vi "AMC Local Process 2.vi"() -> ()   [LabVIEW 2009]
uses:
  vi.lib/NI/AMC/AMC.lvlib
panel:
  in  "Process 1":bool
  out "Process":bool
  out "Status":string
  in  "Local Process":bool
  in  "Exit":bool
  in  "State Variables":cluster{"CurrentFile":path}
  # "Process 2"
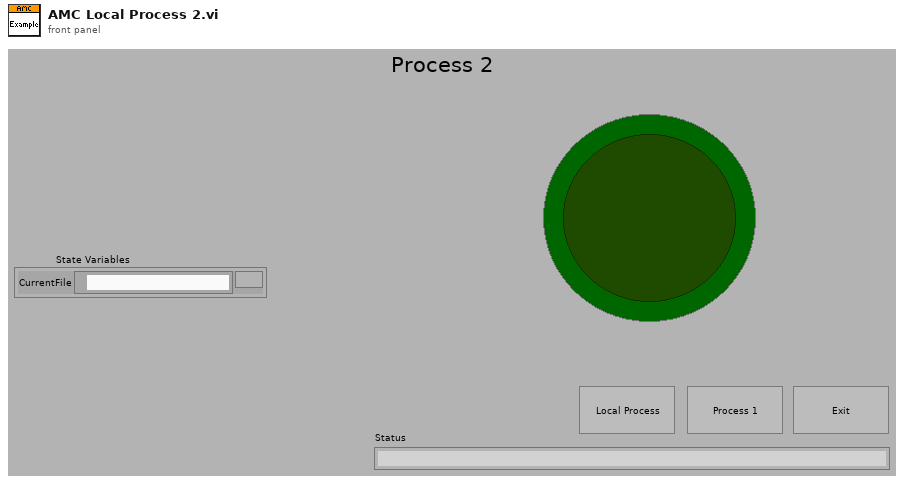
[diagram p1: front panel]
types:
  T1 = typedef "AMC.lvlib/Message Queue.ctl" = refnum<queue>
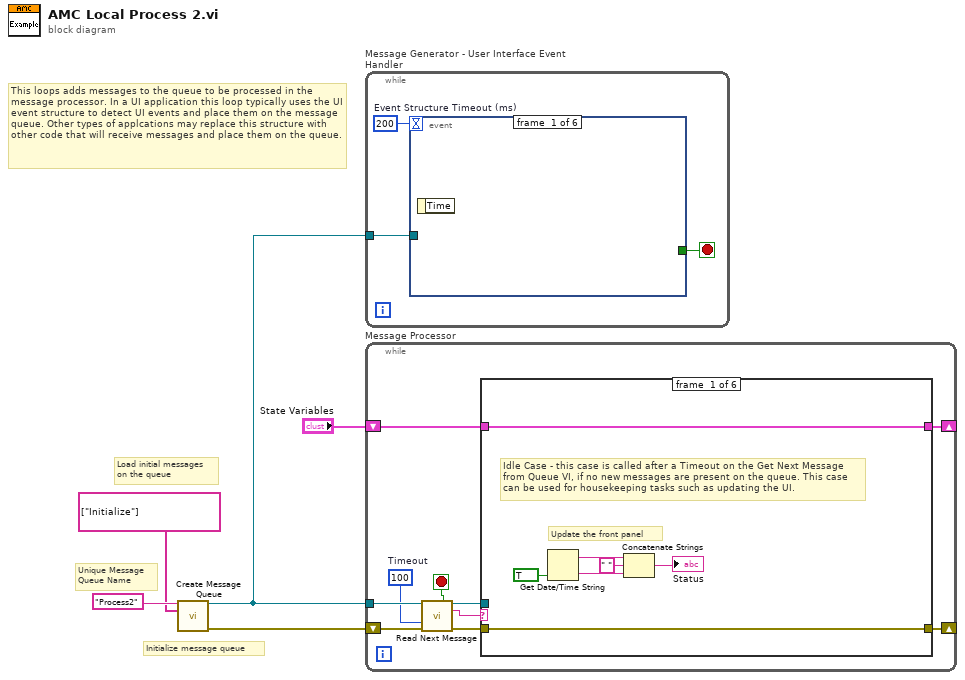
[diagram p0: block diagram]
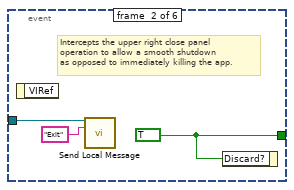
[diagram p2: hidden frame]
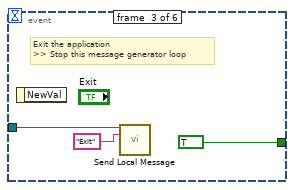
[diagram p3: hidden frame]
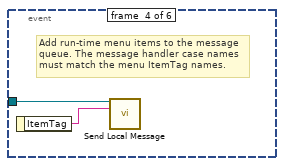
[diagram p4: hidden frame]
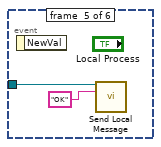
[diagram p5: hidden frame]
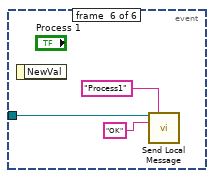
[diagram p6: hidden frame]
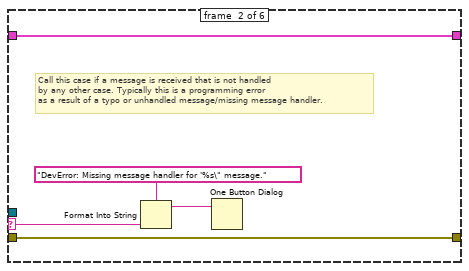
[diagram p7: hidden frame]
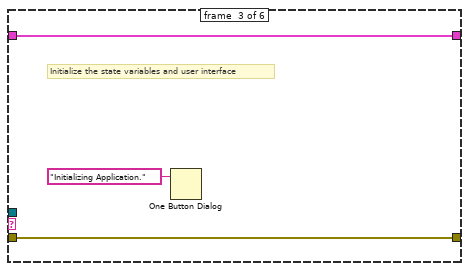
[diagram p8: hidden frame]
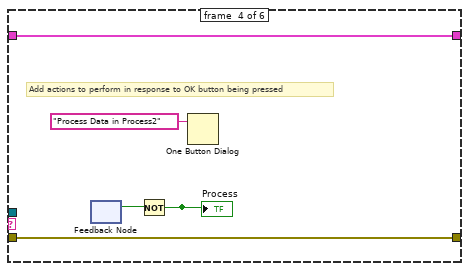
[diagram p9: hidden frame]
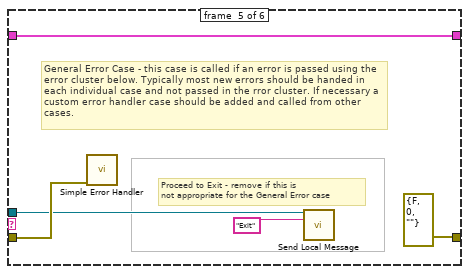
[diagram p10: hidden frame]
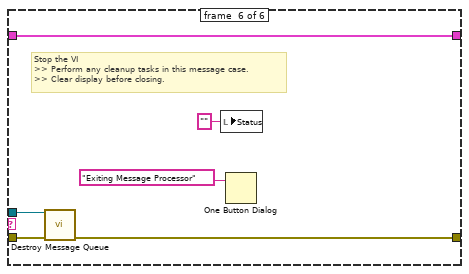
[diagram p11: hidden frame]
diagram:
  # "This loops adds messages to the queue to be processed in the message processor. In a UI application this loop typically uses the UI event structure to detect UI events and place them on the message queue. Other types of applcations may replace this structure with other code that will receive messages and place them on the queue."
  # "Initialize message queue"
  # "Unique Message\nQueue Name"
  # "Load initial messages\non the queue"
  n1 = call "Create Message Queue.vi"("message queue name"="Process2" ("Message queue name (unnamed)"), "initial message names"=string[] ["Initialize"]) -> ("message queue out"=w5:T1, "error out"=w3:errorcluster)  [unwired: 12 in]
  n2 = while "Message Generator - User Interface Event Handler" {
    tunnel: w5 -> [w6]
    stop <- w7 stop-if-true
    w8 = 200  # Event Structure Timeout (ms)
    n3 = event shown="[5] \"Process 1\": Value Change" {
      selector: _ -> [_ _ _ _ _ _]
      dyn-events: _ -> [_ _ _ _ _ _]
      timeout: w8 -> [_ _ _ _ _ _]
      tunnel: [_ w11 TRUE ("Discard?") _ _ _] -> w7
      tunnel: w6 -> [_ w10 w13 w16 w18 w21]
      event #0 {
        n4 = event-data() -> ()  [unwired: 2 out]
      }
      event #1 {
        w11 = TRUE ("Discard?")
        # "Intercepts the upper right close panel\noperation to allow a smooth shutdown\nas opposed to immediately killing the app."
        n5 = event-data() -> ()  [unwired: 2 out]
        n6 = call "Send Local Message.vi"("message queue in"=w10, "message name"="Exit") -> ()  [unwired: 11 in, 3 out]
        n7 = event-data("Discard?"=w11) -> ()  [unwired: 1 in, 1 out]
      }
      event #2 {
        # "Exit the application\n>> Stop this message generator loop"
        n8 = event-data() -> ()  [unwired: 2 out]
        n9 = call "Send Local Message.vi"("message queue in"=w13, "message name"="Exit") -> ()  [unwired: 11 in, 3 out]
      }
      event #3 {
        # "Add run-time menu items to the message\nqueue. The message handler case names must match the menu ItemTag names."
        n10 = event-data() -> ("ItemTag"=w15:string)  [unwired: 1 out]
        n11 = call "Send Local Message.vi"("message queue in"=w16, "message name"=w15) -> ()  [unwired: 11 in, 3 out]
      }
      event #4 {
        n12 = event-data() -> ()  [unwired: 2 out]
        n13 = call "Send Local Message.vi"("message queue in"=w18, "message name"="OK") -> ()  [unwired: 11 in, 3 out]
      }
      event #5 {
        n14 = event-data() -> ()  [unwired: 2 out]
        n15 = call "Send Local Message.vi"("message queue in"=w21, "receiver process (\"\" - local)"="Process1" ("process"), "message name"="OK") -> ()  [unwired: 10 in, 3 out]
      }
    }
  }
  n16 = while "Message Processor" {
    shift-left: w3 -> [w26]
    shift-right: [w27] -> _
    tunnel: w5 -> [w25]
    shift-left: "State Variables" -> [w31]
    shift-right: [w30] -> _
    stop <- w24 stop-if-true
    w22 = 100  # Timeout
    n17 = call "Read Next Message.vi"("message queue in"=w25, "timeout (1 ms)"=w22, "error in"=w26) -> ("exit process?"=w24:bool, "message queue out"=w29:T1, "message name"=w23:string, "error out"=w28:errorcluster)  [unwired: 5 in, 4 out]
    n18 = case shown="\"Initialize\"" w23 {
      selector: w23 -> [_ w41 _ _ _ _]
      tunnel: [w38 w43 w46 w50 w56 w61] -> w30
      tunnel: w31 -> [w38 w43 w46 w50 w56 w61]
      tunnel: w29 -> [_ _ _ _ w53 w58]
      tunnel: w28 -> [w37 w42 w45 w51 w54 w62]
      tunnel: [w37 w42 w45 w51 errorcluster {"status"=FALSE, "code"=0, "source"=""} ("error out") w60] -> w27
      frame #0 {
        # "Update the front panel"
        # "Idle Case - this case is called after a Timeout on the Get Next Message from Queue VI, if no new messages are present on the queue. This case can be used for housekeeping tasks such as updating the UI."
        n19 = Get Date/Time String(want seconds? (F)=TRUE) -> (date string=w36:string, time string=w35:string)  [unwired: 2 out]
        n20 = Concatenate Strings(w36, " " ("string"), w35) -> (→"Status":string)
      }
      frame #1 {
        # "Call this case if a message is received that is not handled \nby any other case. Typically this is a programming error\nas a result of a typo or unhandled message/missing message handler."
        n21 = Format Into String(format string="DevError: Missing message handler for '%s\" message." ("message"), w41) -> (resulting string=w39:string)  [unwired: 2 in, 1 out]
        n22 = One Button Dialog(message=w39) -> ()  [unwired: 2 out]
      }
      frame #2 {
        # "Initialize the state variables and user interface"
        n23 = One Button Dialog(message="Initializing Application.") -> ()  [unwired: 2 out]
      }
      frame #3 {
        # "Add actions to perform in response to OK button being pressed"
        n24 = feedback #1() -> (w47:bool)  [unwired: 1 out]
        n25 = Not(x=w47) -> (.not. x?=w48:bool)
        "Process" <- w48
        n26 = One Button Dialog(message="Process Data in Process2") -> ()  [unwired: 2 out]
      }
      frame #4 {
        # "Proceed to Exit - remove if this is\nnot appropriate for the General Error case"
        # "General Error Case - this case is called if an error is passed using the error cluster below. Typically most new errors should be handed in each individual case and not passed in the rror cluster. If necessary a custom error handler case should be added and called from other cases."
        n27 = call <vilib>:"Simple Error Handler.vi"("error in (no error)"=w54) -> ()  [unwired: 1 in, 8 out]
        n28 = call "Send Local Message.vi"("message queue in"=w53, "message name"="Exit") -> ()  [unwired: 11 in, 3 out]
      }
      frame #5 {
        # "Stop the VI\n>> Perform any cleanup tasks in this message case.\n>> Clear display before closing."
        n29 = call "Destroy Message Queue.vi"("message queue in"=w58, "error in"=w62) -> ("error out"=w60:errorcluster)  [unwired: 11 in, 2 out]
        n30 = local write "Status"("" ("Status")) -> ()
        n31 = One Button Dialog(message="Exiting Message Processor" ("button name (\"OK\")")) -> ()  [unwired: 2 out]
      }
    }
  }
